vi "AFE_SGL_gen.vi"(0 "Inputs":T7, 1 "Gains":T6, 2 "Range":T4={"PLL_PIRad_high"=inf, "PLL_PiRad_low"=inf, "IQcmd_high"=inf, "IQcmd_low"=inf, "IDcmd_high"=inf, "IDcmd_low"=inf, "VDcmd_high"=inf, "VDcmd_low"=inf, "VQmcd_high"=inf, "VQcmd_low"=inf}, 5 "Setpoints":cluster{"VDCLink":sgl, "DirectedIdSetpt":sgl}, 7 "Signals":cluster{"resetPLL":bool, "resetControl":bool}, 9 "input valid":bool=TRUE, 12 "Parameters":T5, 13 "ManualControl":T3) -> (4 "Outputs":T2, 10 "output valid":bool, 14 "feedback signals":cluster{"ready for input":bool}, 15 "Actions":T1)   [LabVIEW 2017]
doc: "This VI is created by the NI LabVIEW 2017 FPGA IP Builder.\n\nProject: AFE.lvproj\nTarget: FPGA Target (sbRIO-9607)/IP Builder\nBuild Specification: AFE_SGL_gen\nDirectives Item: AFE_SGL_src\nTop-Level VI: C:\\PowerElectronicControl\\ActiveFrontEnd\\dev\\IPBuilder\\AFE_SGL_src.vi\n\nQuick Device Utilization Estimate\n--------------------------------------------\nSlice Registers: 5.9% (6288 out of 106400)\nSlice LUTs: 22.8% (12133 out of 53200)\nDSP48s: 13.6% (30 out of 220)\nBlock RAMs: 15.7% (44 out of 280)\n\nQuick Performance Estimate\n--------------------------------------------\nClock rate (MHz): 46.38\nInitiation interval (cycles): 134\nPipeline type: Not pipelined\nMinimum latency: 129\nMaximum latency: 133"
uses:
  <vilib>/rvi/IPIntegrationNode/IPINode_Typedef/niFpgaIPINodeSupportedFamilies.ctl
  <vilib>/rvi/IPIntegrationNode/IPINode_Utilities/niFpgaIPINodeSimCore.vi
  <vilib>/rvi/IPIntegrationNode/IPINode_Xnode/niFpgaIPINode.xnode
  AFE_SGL_gen Support/IPBlockSimFiles/xsim.dir/mF4069A38_topH/xsimk00F7A5BA942A4CB3873FB7E5E25CD33C.dll
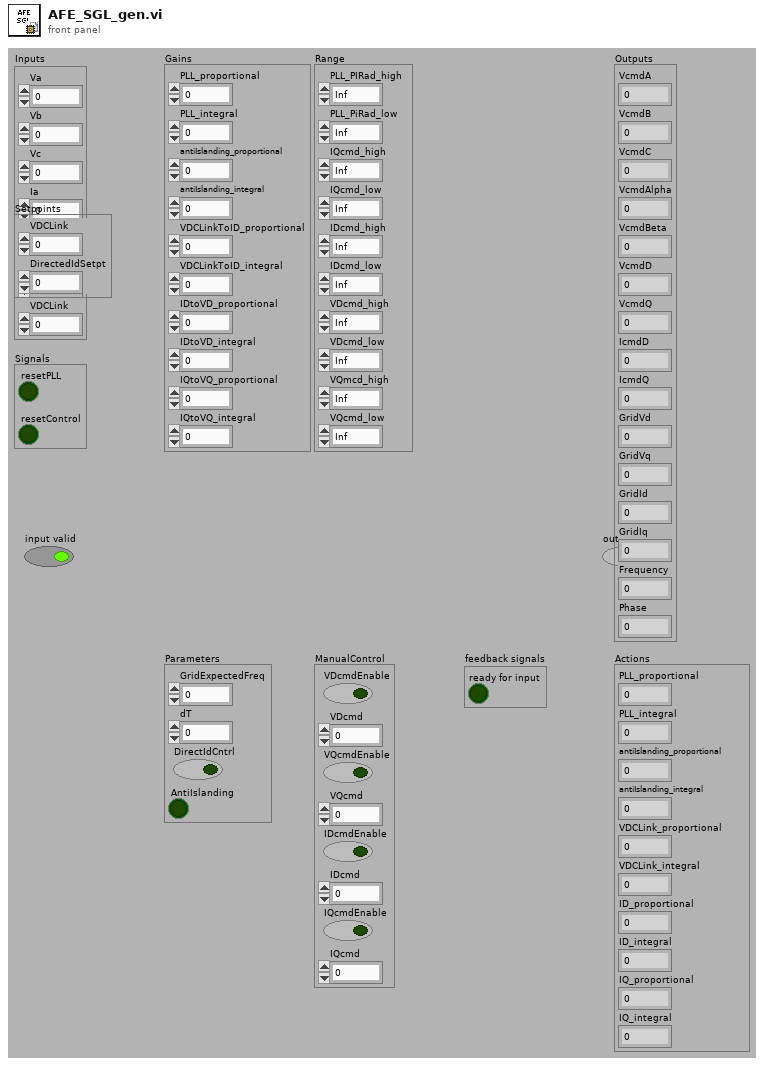
[diagram p1: front panel]
types:
  T1 = cluster{"PLL_proportional":sgl, "PLL_integral":sgl, "antiIslanding_proportional":sgl, "antiIslanding_integral":sgl, "VDCLink_proportional":sgl, "VDCLink_integral":sgl, "ID_proportional":sgl, "ID_integral":sgl, "IQ_proportional":sgl, "IQ_integral":sgl}
  T2 = cluster{"VcmdA":sgl, "VcmdB":sgl, "VcmdC":sgl, "VcmdAlpha":sgl, "VcmdBeta":sgl, "VcmdD":sgl, "VcmdQ":sgl, "IcmdD":sgl, "IcmdQ":sgl, "GridVd":sgl, "GridVq":sgl, "GridId":sgl, "GridIq":sgl, "Frequency":sgl, "Phase":sgl}
  T3 = cluster{"VDcmdEnable":bool, "VDcmd":sgl, "VQcmdEnable":bool, "VQcmd":sgl, "IDcmdEnable":bool, "IDcmd":sgl, "IQcmdEnable":bool, "IQcmd":sgl}
  T4 = cluster{"PLL_PIRad_high":sgl, "PLL_PiRad_low":sgl, "IQcmd_high":sgl, "IQcmd_low":sgl, "IDcmd_high":sgl, "IDcmd_low":sgl, "VDcmd_high":sgl, "VDcmd_low":sgl, "VQmcd_high":sgl, "VQcmd_low":sgl}
  T5 = cluster{"GridExpectedFreq":sgl, "dT":sgl, "DirectIdCntrl":bool, "AntiIslanding":bool}
  T6 = cluster{"PLL_proportional":sgl, "PLL_integral":sgl, "antiIslanding_proportional":sgl, "antiIslanding_integral":sgl, "VDCLinkToID_proportional":sgl, "VDCLinkToID_integral":sgl, "IDtoVD_proportional":sgl, "IDtoVD_integral":sgl, "IQtoVQ_proportional":sgl, "IQtoVQ_integral":sgl}
  T7 = cluster{"Va":sgl, "Vb":sgl, "Vc":sgl, "Ia":sgl, "Ib":sgl, "Ic":sgl, "VDCLink":sgl}
  T8 = cluster{"p_3_e_0":sgl, "p_3_e_1":sgl, "p_3_e_2":sgl, "p_3_e_3":sgl, "p_3_e_4":sgl, "p_3_e_5":sgl, "p_3_e_6":sgl, "p_3_e_7":sgl, "p_3_e_8":sgl, "p_3_e_9":sgl, "p_3_e_10":sgl, "p_3_e_11":sgl, "p_3_e_12":sgl, "p_3_e_13":sgl, "p_3_e_14":sgl}
  T9 = cluster{"p_0_e_0":sgl, "p_0_e_1":sgl, "p_0_e_2":sgl, "p_0_e_3":sgl, "p_0_e_4":sgl, "p_0_e_5":sgl, "p_0_e_6":sgl, "p_0_e_7":sgl, "p_0_e_8":sgl, "p_0_e_9":sgl}
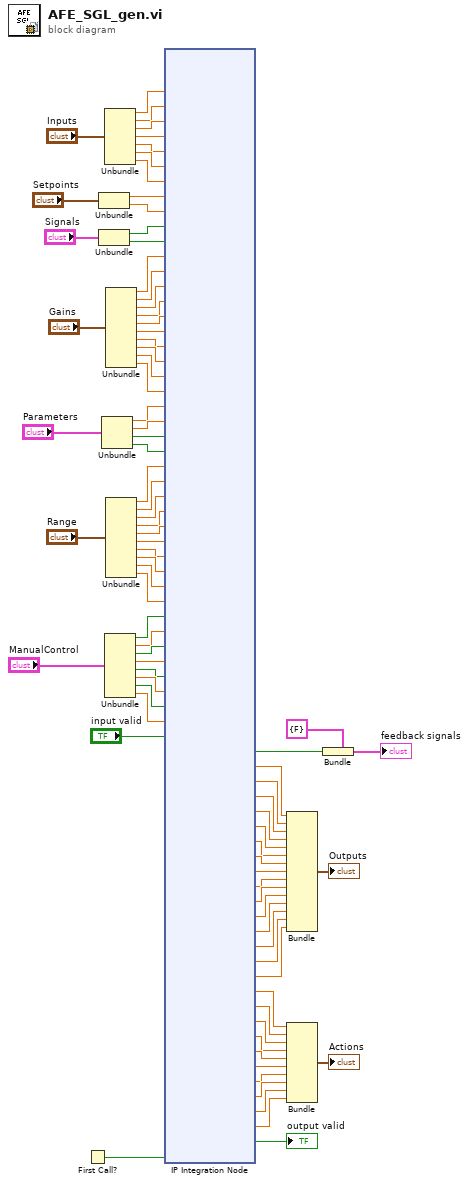
[diagram p0: block diagram]
diagram:
  n1 = First Call?() -> (First Call?: T/F=w83:bool)
  n2 = Unbundle("Setpoints") -> ("VDCLink"=w60:sgl, "DirectedIdSetpt"=w61:sgl)
  n3 = Unbundle("Signals") -> ("resetPLL"=w58:bool, "resetControl"=w59:bool)
  n4 = Unbundle("Parameters") -> ("GridExpectedFreq"=w44:sgl, "dT"=w45:sgl, "DirectIdCntrl"=w46:bool, "AntiIslanding"=w47:bool)
  n5 = Unbundle("Inputs") -> ("Va"=w62:sgl, "Vb"=w63:sgl, "Vc"=w64:sgl, "Ia"=w65:sgl, "Ib"=w66:sgl, "Ic"=w67:sgl, "VDCLink"=w68:sgl)
  n6 = Unbundle("ManualControl") -> ("VDcmdEnable"=w26:bool, "VDcmd"=w27:sgl, "VQcmdEnable"=w28:bool, "VQcmd"=w29:sgl, "IDcmdEnable"=w30:bool, "IDcmd"=w31:sgl, "IQcmdEnable"=w32:bool, "IQcmd"=w33:sgl)
  n7 = Unbundle("Gains") -> ("PLL_proportional"=w48:sgl, "PLL_integral"=w49:sgl, "antiIslanding_proportional"=w50:sgl, "antiIslanding_integral"=w51:sgl, "VDCLinkToID_proportional"=w52:sgl, "VDCLinkToID_integral"=w53:sgl, "IDtoVD_proportional"=w54:sgl, "IDtoVD_integral"=w55:sgl, "IQtoVQ_proportional"=w56:sgl, "IQtoVQ_integral"=w57:sgl)
  n8 = Unbundle("Range") -> ("PLL_PIRad_high"=w34:sgl, "PLL_PiRad_low"=w35:sgl, "IQcmd_high"=w36:sgl, "IQcmd_low"=w37:sgl, "IDcmd_high"=w38:sgl, "IDcmd_low"=w39:sgl, "VDcmd_high"=w40:sgl, "VDcmd_low"=w41:sgl, "VQmcd_high"=w42:sgl, "VQcmd_low"=w43:sgl)
  n9 = xnode "IP Integration Node"("p_11_e_0"=w62, "p_11_e_1"=w63, "p_11_e_2"=w64, "p_11_e_3"=w65, "p_11_e_4"=w66, "p_11_e_5"=w67, "p_11_e_6"=w68, "p_10_e_0"=w60, "p_10_e_1"=w61, "p_9_e_0"=w58, "p_9_e_1"=w59, "p_7_e_0"=w48, "p_7_e_1"=w49, "p_7_e_2"=w50, "p_7_e_3"=w51, "p_7_e_4"=w52, "p_7_e_5"=w53, "p_7_e_6"=w54, "p_7_e_7"=w55, "p_7_e_8"=w56, "p_7_e_9"=w57, "p_6_e_0"=w44, "p_6_e_1"=w45, "p_6_e_2"=w46, "p_6_e_3"=w47, "p_5_e_0"=w34, "p_5_e_1"=w35, "p_5_e_2"=w36, "p_5_e_3"=w37, "p_5_e_4"=w38, "p_5_e_5"=w39, "p_5_e_6"=w40, "p_5_e_7"=w41, "p_5_e_8"=w42, "p_5_e_9"=w43, "p_4_e_0"=w26, "p_4_e_1"=w27, "p_4_e_2"=w28, "p_4_e_3"=w29, "p_4_e_4"=w30, "p_4_e_5"=w31, "p_4_e_6"=w32, "p_4_e_7"=w33, "input_valid"="input valid", "first_call"=w83) -> ("ready_for_input"=w80:bool, "p_3_e_0"=w11:sgl, "p_3_e_1"=w12:sgl, "p_3_e_2"=w13:sgl, "p_3_e_3"=w14:sgl, "p_3_e_4"=w15:sgl, "p_3_e_5"=w16:sgl, "p_3_e_6"=w17:sgl, "p_3_e_7"=w18:sgl, "p_3_e_8"=w19:sgl, "p_3_e_9"=w20:sgl, "p_3_e_10"=w21:sgl, "p_3_e_11"=w22:sgl, "p_3_e_12"=w23:sgl, "p_3_e_13"=w24:sgl, "p_3_e_14"=w25:sgl, "p_0_e_0"=w1:sgl, "p_0_e_1"=w2:sgl, "p_0_e_2"=w3:sgl, "p_0_e_3"=w4:sgl, "p_0_e_4"=w5:sgl, "p_0_e_5"=w6:sgl, "p_0_e_6"=w7:sgl, "p_0_e_7"=w8:sgl, "p_0_e_8"=w9:sgl, "p_0_e_9"=w10:sgl, "output_valid"=→"output valid":bool)  [unwired: 2 in]
  n10 = Bundle("p_3_e_0"=w11, "p_3_e_1"=w12, "p_3_e_2"=w13, "p_3_e_3"=w14, "p_3_e_4"=w15, "p_3_e_5"=w16, "p_3_e_6"=w17, "p_3_e_7"=w18, "p_3_e_8"=w19, "p_3_e_9"=w20, "p_3_e_10"=w21, "p_3_e_11"=w22, "p_3_e_12"=w23, "p_3_e_13"=w24, "p_3_e_14"=w25) -> (→"Outputs":T8)  [unwired: 1 in]
  n11 = Bundle("p_0_e_0"=w1, "p_0_e_1"=w2, "p_0_e_2"=w3, "p_0_e_3"=w4, "p_0_e_4"=w5, "p_0_e_5"=w6, "p_0_e_6"=w7, "p_0_e_7"=w8, "p_0_e_8"=w9, "p_0_e_9"=w10) -> (→"Actions":T9)  [unwired: 1 in]
  n12 = Bundle ("Bundle_feedback")(cluster=cluster{"ready for input":bool} {"ready for input"=FALSE}, "ready for input"=w80) -> (→"feedback signals":cluster{"ready for input":bool})
